vi "InvertDirection.vi"(1 "did we just start?":bool, 5 "Direction":dbl, 7 "Target Position [deg]":dbl, 9 "Position [deg]":dbl, 11 "Starting position":dbl format="%#_13g", 12 "HalfOfHapticBumpLength":dbl) -> (6 "Direction":dbl, 14 "Difference at start(position and target)":dbl)   [LabVIEW 2019]
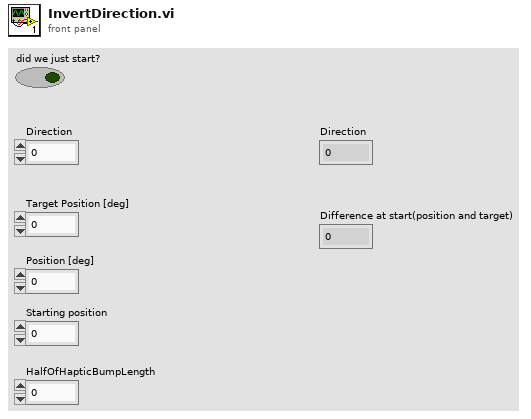
[diagram p1: front panel]
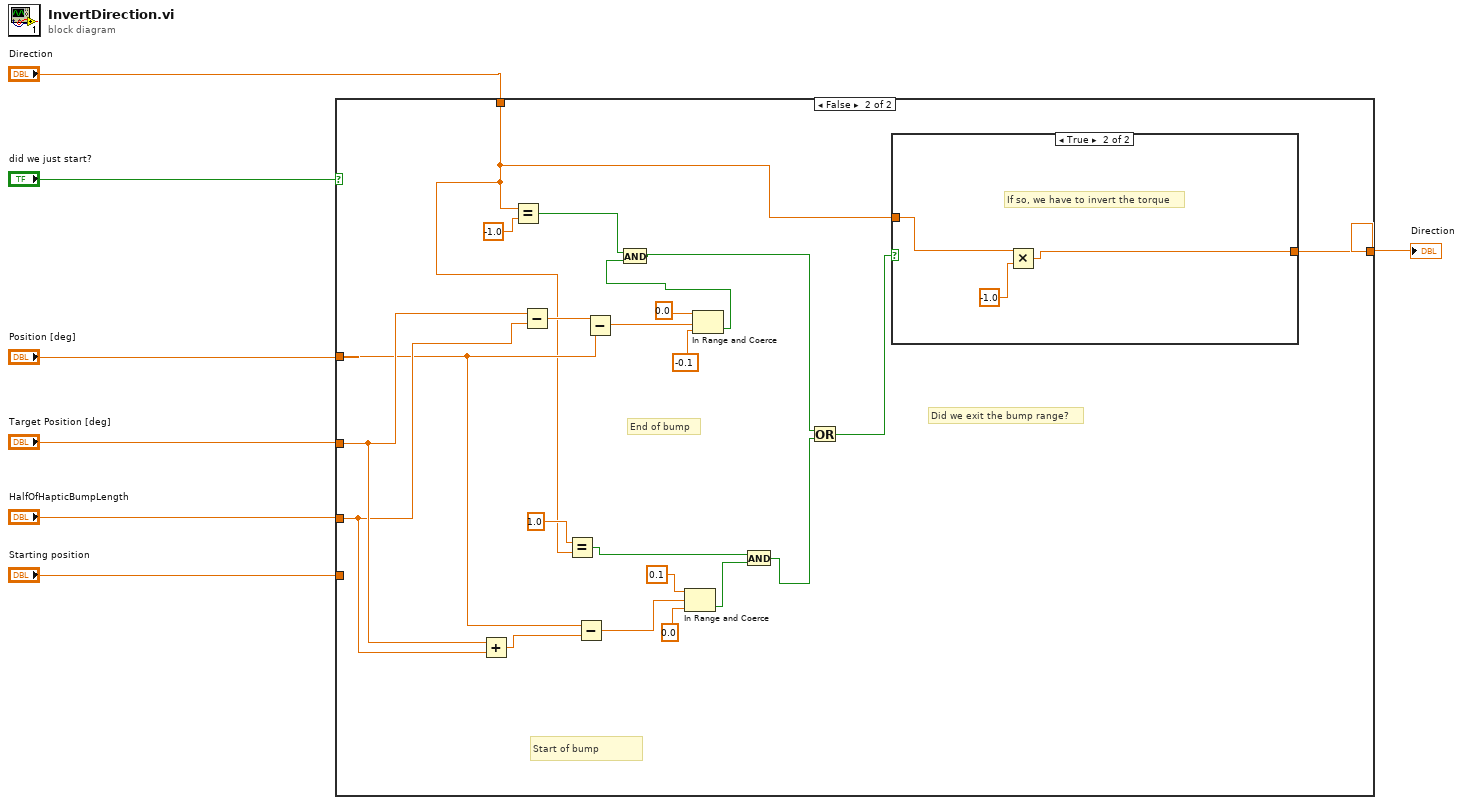
[diagram p0: block diagram]
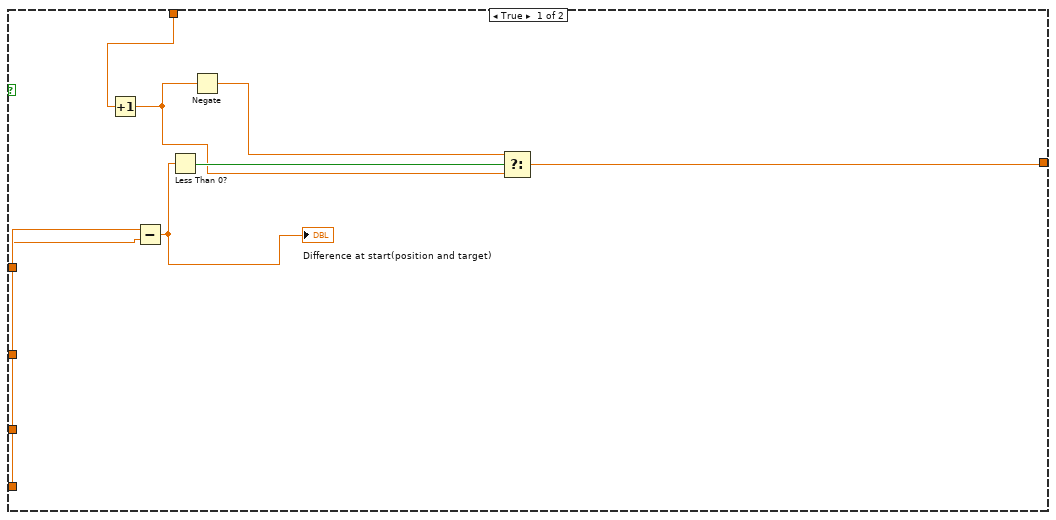
[diagram p2: hidden frame]
diagram:
  n1 = case shown="False" "did we just start?" {
    tunnel: "Position [deg]" -> [_ w27]
    tunnel: "Direction" -> [w12 w19]
    tunnel: [w13 w35] -> w1
    tunnel: "Target Position [deg]" -> [w10 w29]
    tunnel: "HalfOfHapticBumpLength" -> [_ w28]
    tunnel: "Starting position" -> [w8 _]
    frame True {
      n2 = Increment(x=w12) -> (x+1=w11:dbl)
      n3 = Subtract(x=w10, y=w8) -> (x-y=w9:dbl)
      "Difference at start(position and target)" <- w9
      n4 = Less Than 0?(x=w9) -> (x < 0?=w15:bool)
      n5 = Negate(x=w11) -> (-x=w14:dbl)
      n6 = Select(t=w14, s=w15, f=w11) -> (s? t:f=w13:dbl)
    }
    frame False {
      # "Did we exit the bump range?"
      # "End of bump"
      # "Start of bump"
      n7 = Add(x=w29, y=w28) -> (x+y=w26:dbl)
      n8 = Equal?(x=w19, y=-1.0) -> (x = y?=w36:bool)
      n9 = Subtract(x=w29, y=w28) -> (x-y=w37:dbl)
      n10 = Equal?(x=1.0, y=w19) -> (x = y?=w21:bool)
      n11 = Subtract(x=w27, y=w26) -> (x-y=w25:dbl)
      n12 = Subtract(x=w37, y=w27) -> (x-y=w30:dbl)
      n13 = In Range and Coerce(upper limit=0.1, x=w25, lower limit=0.0) -> (In Range?=w20:bool)  [unwired: 1 out]
      n14 = In Range and Coerce(upper limit=0.0, x=w30, lower limit=-0.1) -> (In Range?=w33:bool)  [unwired: 1 out]
      n15 = And(x=w36, y=w33) -> (x .and. y?=w17:bool)
      n16 = And(x=w21, y=w20) -> (x .and. y?=w18:bool)
      n17 = Or(x=w17, y=w18) -> (x .or. y?=w16:bool)
      n18 = case shown="True" w16 {
        tunnel: w19 -> [w38 w40]
        tunnel: [w38 w41] -> w35
        frame False {
        }
        frame True {
          # "If so, we have to invert the torque"
          n19 = Multiply(x=w40, y=-1.0) -> (x*y=w41:dbl)
        }
      }
    }
  }
  "Direction" <- w1
